vi "write_attributes.vi"(8 "error in (no error)":errorcluster, 10 "attributes":T1, 11 "GaussianProcessRegressor in":refnum<class "GaussianProcessRegressor.lvclass">) -> (0 "error out":errorcluster, 3 "GaussianProcessRegressor out":refnum<class "GaussianProcessRegressor.lvclass">)   [LabVIEW 2020, in "GaussianProcessRegressor.lvclass"]
uses:
  GaussianProcessRegressor.lvclass
  Controls/gaussian_process_regressor_attributes.ctl
  GaussianProcessRegressor.lvclass/GaussianProcessRegressor.ctl
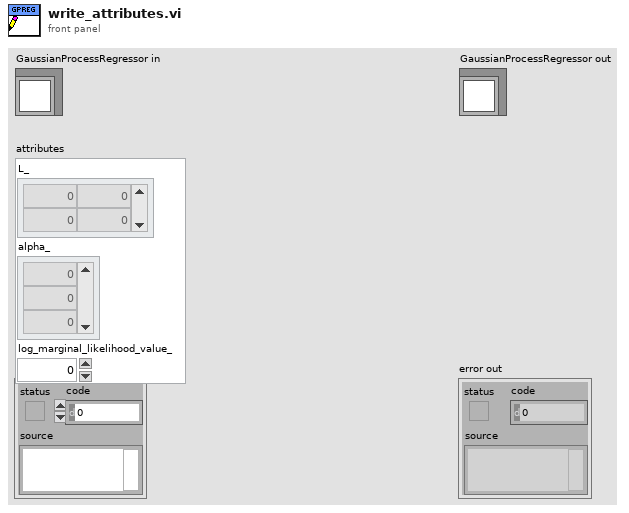
[diagram p1: front panel]
types:
  T1 = typedef "gaussian_process_regressor_attributes.ctl" = cluster{"L_":dbl[][], "alpha_":dbl[], "log_marginal_likelihood_value_":dbl}
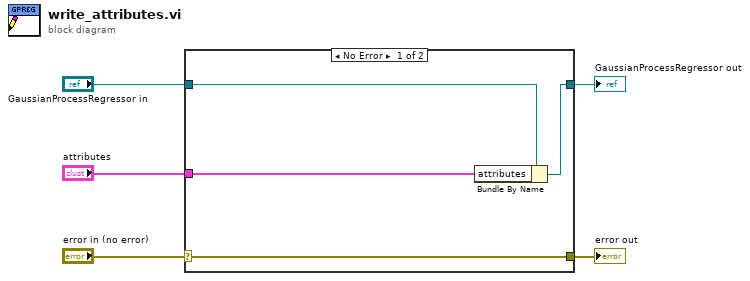
[diagram p0: block diagram]
diagram:
  n1 = case shown="No Error" "error in (no error)" {
    selector: "error in (no error)" -> [w9 w10]
    tunnel: [w9 w10] -> w4
    tunnel: [w7 w11] -> w2
    tunnel: "GaussianProcessRegressor in" -> [w8 w11]
    tunnel: "attributes" -> [w6 _]
    frame No Error {
      n2 = Bundle By Name(cluster=w8, "attributes"=w6) -> (w7:refnum<class "GaussianProcessRegressor.lvclass">)
    }
    frame Error {
    }
  }
  "error out" <- w4
  "GaussianProcessRegressor out" <- w2
